vi "Configure Auto Zero Mode [AZ].vi"(8 "error in (no error)":errorcluster, 10 "auto zero mode (Off)":i32(ring) items=["On"=1, "Off"=0, "Once"=2], 11 "CS++DMM in":refnum<class "CS++DMM.lvclass">) -> (0 "error out":errorcluster, 3 "CS++DMM out":refnum<class "CS++DMM.lvclass">)   [LabVIEW 2015, in "CS++DMM.lvlib" / "CS++DMM.lvclass"]
doc: "This VI configures the auto zero mode of the DMM.\n\nNote:\n\n(1) This VI is part of the IviDmmAutoZero [AZ] extension group."
uses:
  CS++DMM.lvclass
  CSPP_Core/Classes/CS++ProcessVariables/ProcessVariable/PV.lvclass
  PV-Enum.ctl
  CSPP_Core/Classes/CS++ProcessVariables/ProcessVariable/PV.lvclass/PV.ctl
  CS++DMM.lvclass/CS++DMM.ctl
  CSPP_Core/Classes/CS++ProcessVariables/ProcessVariable/Write Data.vi
  CSPP_Core/Classes/CS++ProcessVariables/ProcessVariable/Write Timestamp.vi
  CSPP_Core/Classes/CS++ProcessVariables/ProcessVariable/Write Quality.vi
  CSPP_Core/Classes/CS++ProcessVariables/ProcessVariable/Write status.vi
  CSPP_Core/Classes/CS++ProcessVariables/PVConnection/PVConnection.lvclass
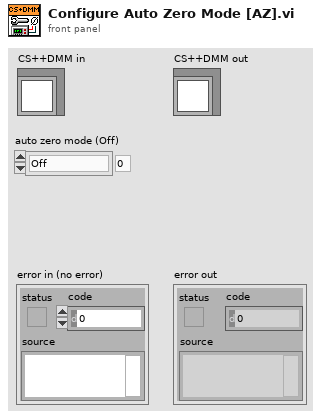
[diagram p1: front panel]
types:
  T1 = typedef "CS++DMM.lvlib/CS++DMM.lvclass/PV-Enum.ctl" = enum16{"AbsoluteResolution", "ACMaxFrequency", "ACMinFrequency", "ActualRange", "Alpha", "ApertureTime", "FixedReferenceJunction", "FrequencyVoltageRange", "PowerLineFrequency", "Range", "Reading", "Resistance", "SampleInterval", "TriggerDelay", "ApertureTimeUnit", "AutoZeroMode", "MeasCompleteDestination", "MeasurementFunction", "ReferenceJunctionType", "SampleCount", "SampleTrigger", "ThermocoupleType", "TranducerType", "TriggerCount", "TriggerSlope", "TriggerSource", "MPReading", "IsOverRange"}
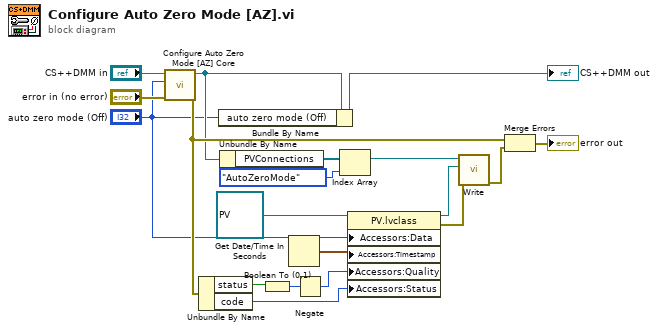
[diagram p0: block diagram]
diagram:
  n1 = call-dynamic "Configure Auto Zero Mode [AZ] Core.vi"("error in (no error)"="error in (no error)", "auto zero mode (Off)"="auto zero mode (Off)", "CS++DMM in"="CS++DMM in") -> ("error out"=w7:errorcluster, "CS++DMM out"=w5:refnum<class "CS++DMM.lvclass">)  [unwired: 7 in]
  n2 = Unbundle By Name(w7) -> ("status"=w16:bool, "code"=w13:i32)
  n3 = Bundle By Name(cluster=w5, "auto zero mode (Off)"="auto zero mode (Off)") -> (→"CS++DMM out":refnum<class "CS++DMM.lvclass">)
  n4 = Unbundle By Name(w5) -> ("PVConnections"=w9:refnum<class "PVConnection.lvclass">[])
  n5 = Boolean To (0,1)(Boolean=w16) -> (0, 1=w15:i16)
  n6 = Get Date/Time In Seconds() -> (seconds since 1Jan1904=w12:timestamp)
  n7 = Negate(x=w15) -> (-x=w14:i16)
  n8 = Index Array(array=w9, index=PV-Enum."AutoZeroMode" ("PV-Enum")) -> (element=w2:refnum<class "PVConnection.lvclass">)
  n9 = property class="PV.lvclass"(reference=refnum<class "PV.lvclass"> refnum ("CS++ProcessVariables.lvlib:PV.lvclass"), "Accessors:Data"="auto zero mode (Off)", "Accessors:Timestamp"=w12, "Accessors:Quality"=w14, "Accessors:Status"=w13) -> (reference out=w10:refnum<class "PV.lvclass">, error out=w11:errorcluster)  [unwired: 1 in]
  n10 = call "Write.vi"("error in (no error)"=w11, "PV"=w10, "PVConnection in"=w2) -> ("error out"=w8:errorcluster)  [unwired: 7 in, 1 out]
  n11 = Merge Errors(w7, w8) -> (→"error out":errorcluster)
